vi "string motor msg to array of double speeds.vi"(1 "Length of individual speed command (default: 6) (including sign)":i32=6, 2 "read buffer":string) -> (0 "All speeds array (double)":dbl[](array[numeric]))   [LabVIEW 2018]
uses:
  sabertooth-packetized-control/code/package/variables/Sabertooths in use gvar.vi
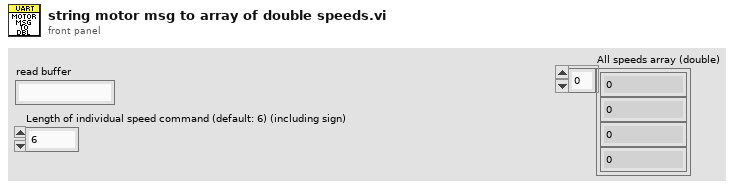
[diagram p1: front panel]
types:
  T1 = typedef "All Addresses.ctl" = u8[]
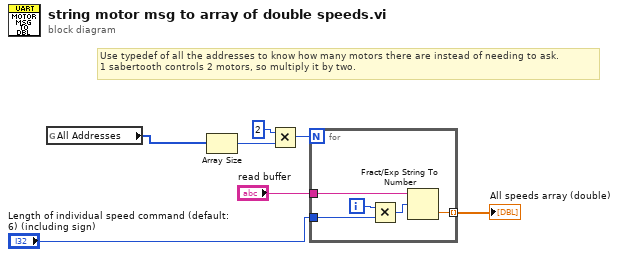
[diagram p0: block diagram]
diagram:
  # "Use typedef of all the addresses to know how many motors there are instead of needing to ask.\n1 sabertooth controls 2 motors, so multiply it by two."
  n1 = global read "Sabertooths in use gvar.vi" "All Addresses"() -> (w1:T1)
  n2 = Array Size(array=w1) -> (size(s)=w4:i32)
  n3 = Multiply(x=2, y=w4) -> (x*y=w3:i32)
  n4 = for {
    N: w3 -> [_]
    tunnel: [w12] -> w7 mode=indexing
    tunnel: "read buffer" -> [w10]
    tunnel: "Length of individual speed command (default: 6) (including sign)" -> [w8]
    i -> [w9]
    n5 = Multiply(x=w9, y=w8) -> (x*y=w11:i32)
    n6 = Fract/Exp String To Number(string=w10, offset=w11) -> (number=w12:dbl)  [unwired: 2 in, 1 out]
  }
  "All speeds array (double)" <- w7
